vi "Write Send Status String Msg.vi"(10 "Test.lvlib:Send Status String Msg.lvclass":refnum<class "Status String Msg.lvclass">, 11 "Test in":refnum<class "Test.lvclass">) -> (3 "Test out":refnum<class "Test.lvclass">)   [LabVIEW 2017, in "Test.lvlib" / "Test.lvclass"]
uses:
  Test.lvclass
  Test Messages/Send Status String Msg/Status String Msg.lvclass
  Test.lvclass/Test.ctl
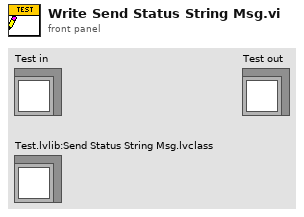
[diagram p1: front panel]
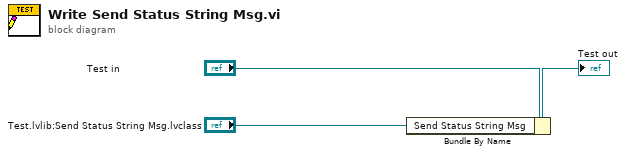
[diagram p0: block diagram]
diagram:
  n1 = Bundle By Name(cluster="Test in", "Send Status String Msg"="Test.lvlib:Send Status String Msg.lvclass") -> (→"Test out":refnum<class "Test.lvclass">)
